vi "Get SMO Address.vi"(8 "error in (no error)":errorcluster, 11 "Inst.Magneto in":refnum<class "Inst.Magneto.lvclass">) -> (0 "error out":errorcluster, 2 "SMO Address":string, 3 "Inst.Magneto out":refnum<class "Inst.Magneto.lvclass">)   [LabVIEW 2019, in "Inst.Magneto.lvclass"]
uses:
  Inst.Magneto.lvclass
  <userlib>/Levylab/Instrument Framework/Instrument Types/VSource/Instrument.VSource.lvclass
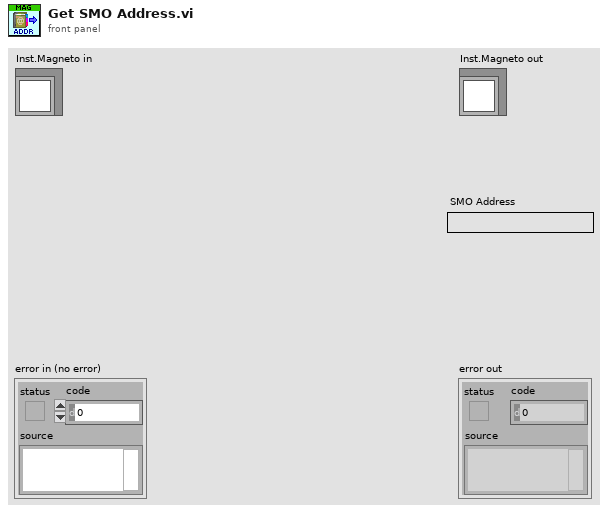
[diagram p1: front panel]
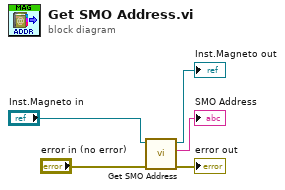
[diagram p0: block diagram]
diagram:
  n1 = call-parent "Get SMO Address.vi"("error in (no error)"="error in (no error)", "Instrument in"="Inst.Magneto in") -> ("error out"=→"error out":errorcluster, "SMO Address"=→"SMO Address":string, "Instrument out"=→"Inst.Magneto out":refnum<class "Inst.Magneto.lvclass">)  [unwired: 7 in]
